vi "FPGA_AIReadAccumulatorCenter.vi"(8 "error in (no error)":errorcluster, 10 "Channel":T1=enum."AI 1", 11 "AI Reference in":T2) -> (0 "error out":errorcluster, 1 "Center":i32, 3 "AI Reference out":T2)   [LabVIEW 2017]
uses:
  <vilib>/Rock Robotics/SystemInterfaces/AI/FPGA_AIDevRef.ctl
  <vilib>/Rock Robotics/SystemInterfaces/AI/FPGA_AIChannel.ctl
  <vilib>/Rock Robotics/SystemInterfaces/System/FPGA_SystemFPGA Ref Global.vi
  <vilib>/Utility/error.llb/Error Cluster From Error Code.vi
  <vilib>/rvi/errors/niLvFpgaAdjustHostInterfaceError.vi
  <vilib>/rvi/interface/nirviReadWriteControl/nirviReadWriteControl.xnode
  <vilib>/Rock Robotics/SystemInterfaces/System/FPGA_SystemFRC FPGA Ref.ctl
  <vilib>/rvi/interface/Simulation/niFpgaSimulationCallBeginRW.vi
  NiFpgaLv.dll
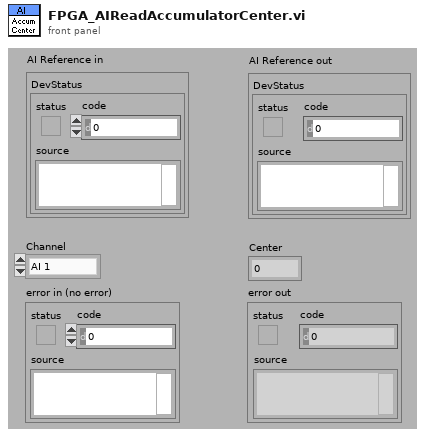
[diagram p1: front panel]
types:
  T1 = typedef "FPGA_AIChannel.ctl" = enum8{"AI 0", "AI 1", "AI 2", "AI 3", "AI MXP 0", "AI MXP 1", "AI MXP 2", "AI MXP 3", "Invalid"}
  T2 = typedef "FPGA_AIDevRef.ctl" = cluster{"DevStatus":errorcluster}
  T3 = typedef "FPGA_SystemFRC FPGA Ref.ctl" = refnum<k20>
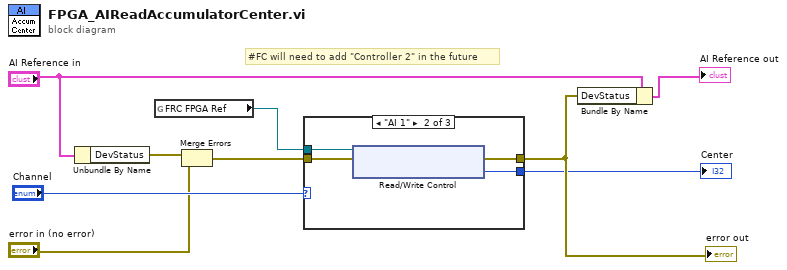
[diagram p0: block diagram]
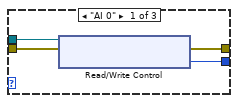
[diagram p2: hidden frame]
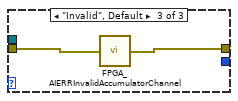
[diagram p3: hidden frame]
diagram:
  # "#FC will need to add \"Controller 2\" in the future"
  n1 = Unbundle By Name("AI Reference in") -> ("DevStatus"=w3:errorcluster)
  n2 = global read "FPGA_SystemFPGA Ref Global.vi" "FRC FPGA Ref"() -> (w4:T3)
  n3 = Merge Errors(w3, "error in (no error)") -> (w2:errorcluster)
  n4 = case shown="\"AI 1\"" "Channel" {
    tunnel: w2 -> [w11 w15 w19]
    tunnel: [w13 w16 w18] -> w7
    tunnel: [w12 w17 _] -> w6
    tunnel: w4 -> [w10 w14 _]
    frame "AI 0" {
      n5 = xnode "Read/Write Control"("FPGA VI Reference In"=w10, "error in"=w11) -> ("error out"=w13:errorcluster, "Accumulator0.Center"=w12:i32)  [unwired: 1 out]
    }
    frame "AI 1" {
      n6 = xnode "Read/Write Control"("FPGA VI Reference In"=w14, "error in"=w15) -> ("error out"=w16:errorcluster, "Accumulator1.Center"=w17:i32)  [unwired: 1 out]
    }
    frame "Invalid", Default {
      n7 = call <vilib>:"FPGA_AIERRInvalidAccumulatorChannel.vi"("error in (no error)"=w19) -> ("error out"=w18:errorcluster)
    }
  }
  "error out" <- w7
  "Center" <- w6
  n8 = Bundle By Name(cluster="AI Reference in", "DevStatus"=w7) -> (→"AI Reference out":T2)
